vi "Get default PCM configuration_Copy.vi"(11 "PCM Interfaces":T6) -> (2 "Frame Sync Clock Control":T1={"Frame Length"=64, "Frame Sync Pulse Width"=32, "Bit Clock Edge  Sync"=enum."Falling"}, 3 "PCM Data Configuration":T3={"Frame Sync Edge for Channel 0"=enum."Falling", "Channel Count Per Frame"=2, "Channel Length"=32, "Bit Depth"=24, "Channel 0 Offset"=1, "Endianness"=enum."MSB First", "Data Justification"=enum."Left Justified"})   [LabVIEW 2021, in "Audio ADC Shared.lvlib"]
uses:
  Audio ADC Shared.lvlib
  controls/PCM Interface Type_Copy.ctl
  <vilib>/PDM Acquisition Toolkit/shared/controls/PCM Data Format Configuration.ctl
  <vilib>/PDM Acquisition Toolkit/shared/controls/Digital Edge.ctl
  <vilib>/PDM Acquisition Toolkit/shared/controls/PCM Bit Endianness.ctl
  <vilib>/PDM Acquisition Toolkit/shared/controls/PCM Data Justification.ctl
  <vilib>/PDM Acquisition Toolkit/shared/controls/PCM Frame Sync Control.ctl
  <vilib>/PDM Acquisition Toolkit/shared/PDM Shared.lvlib
  controls/Audio ADC Controls.lvlib
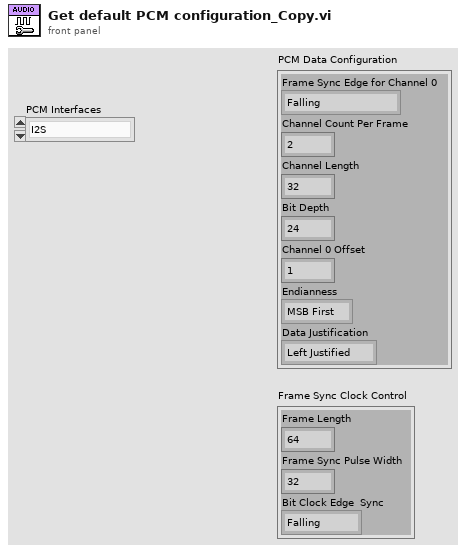
[diagram p1: front panel]
types:
  T1 = typedef "PDM Shared.lvlib/PCM Frame Sync Control.ctl" = cluster{"Frame Length":u16, "Frame Sync Pulse Width":u16, "Bit Clock Edge  Sync":T2}
  T2 = typedef "PDM Shared.lvlib/Digital Edge.ctl" = enum8{"Rising", "Falling"}
  T3 = typedef "PDM Shared.lvlib/PCM Data Format Configuration.ctl" = cluster{"Frame Sync Edge for Channel 0":T2, "Channel Count Per Frame":u8, "Channel Length":u16, "Bit Depth":u8, "Channel 0 Offset":u16, "Endianness":T4, "Data Justification":T5}
  T4 = typedef "PDM Shared.lvlib/PCM Bit Endianness.ctl" = enum16{"MSB First", "LSB First"}
  T5 = typedef "PDM Shared.lvlib/PCM Data Justification.ctl" = enum16{"Left Justified", "Right Justified"}
  T6 = typedef "Audio ADC Controls.lvlib/PCM Interface Type_Copy.ctl" = enum16{"I2S", "Left Justified", "Right Justified", "TDM 4 Channel", "TDM 6 Channel", "TDM 8 Channel", "DSP mode", "DSP mode with 1 bit delay", "PCM Short Frame", "PCM Long Frame"}
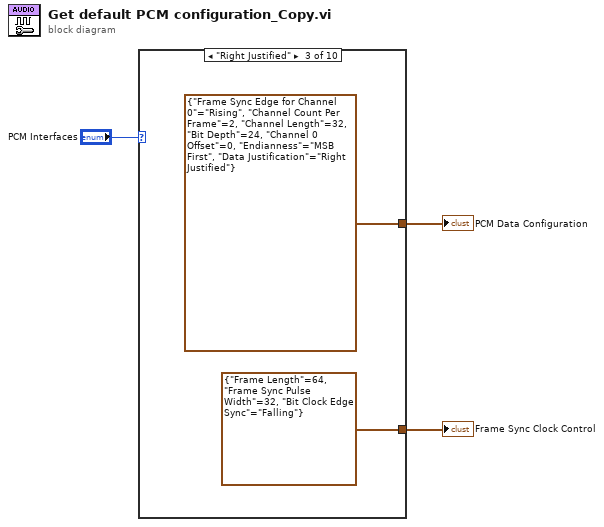
[diagram p0: block diagram]
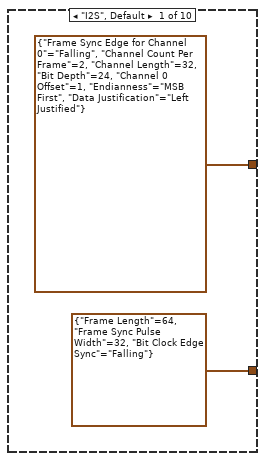
[diagram p2: hidden frame]
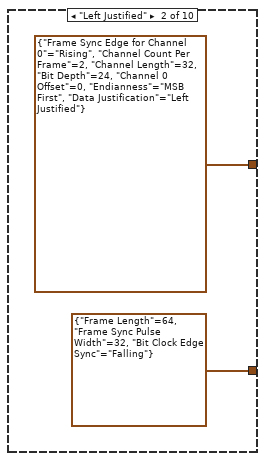
[diagram p3: hidden frame]
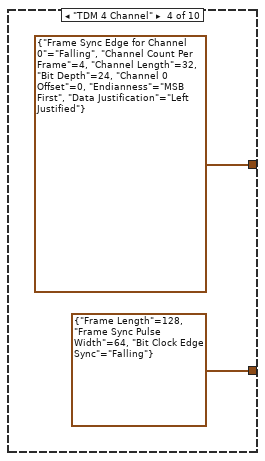
[diagram p4: hidden frame]
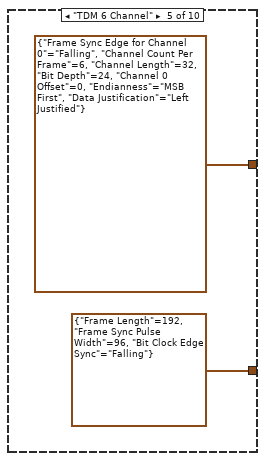
[diagram p5: hidden frame]
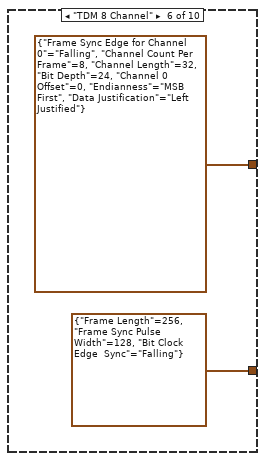
[diagram p6: hidden frame]
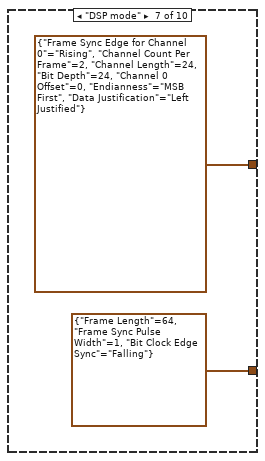
[diagram p7: hidden frame]
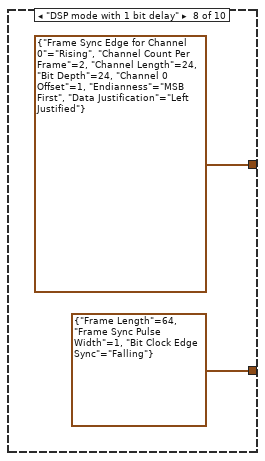
[diagram p8: hidden frame]
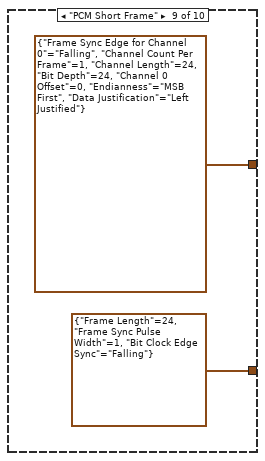
[diagram p9: hidden frame]
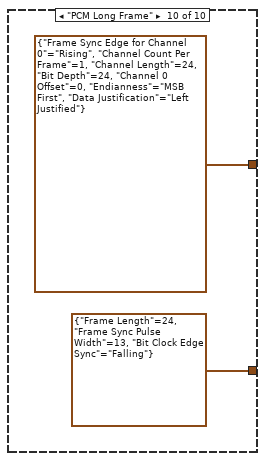
[diagram p10: hidden frame]
diagram:
  n1 = case shown="\"Right Justified\"" "PCM Interfaces" {
    tunnel: [T3 {"Frame Sync Edge for Channel 0"=enum."Falling", "Channel Count Per Frame"=2, "Channel Length"=32, "Bit Depth"=24, "Channel 0 Offset"=1, "Endianness"=enum."MSB First", "Data Justification"=enum."Left Justified"} ("PCM Data Configuration") T3 {"Frame Sync Edge for Channel 0"=enum."Rising", "Channel Count Per Frame"=2, "Channel Length"=32, "Bit Depth"=24, "Channel 0 Offset"=0, "Endianness"=enum."MSB First", "Data Justification"=enum."Left Justified"} ("PCM Data Configuration") T3 {"Frame Sync Edge for Channel 0"=enum."Rising", "Channel Count Per Frame"=2, "Channel Length"=32, "Bit Depth"=24, "Channel 0 Offset"=0, "Endianness"=enum."MSB First", "Data Justification"=enum."Right Justified"} ("PCM Data Configuration") T3 {"Frame Sync Edge for Channel 0"=enum."Falling", "Channel Count Per Frame"=4, "Channel Length"=32, "Bit Depth"=24, "Channel 0 Offset"=0, "Endianness"=enum."MSB First", "Data Justification"=enum."Left Justified"} ("PCM Data Configuration") T3 {"Frame Sync Edge for Channel 0"=enum."Falling", "Channel Count Per Frame"=6, "Channel Length"=32, "Bit Depth"=24, "Channel 0 Offset"=0, "Endianness"=enum."MSB First", "Data Justification"=enum."Left Justified"} ("PCM Data Configuration") T3 {"Frame Sync Edge for Channel 0"=enum."Falling", "Channel Count Per Frame"=8, "Channel Length"=32, "Bit Depth"=24, "Channel 0 Offset"=0, "Endianness"=enum."MSB First", "Data Justification"=enum."Left Justified"} ("PCM Data Configuration") T3 {"Frame Sync Edge for Channel 0"=enum."Rising", "Channel Count Per Frame"=2, "Channel Length"=24, "Bit Depth"=24, "Channel 0 Offset"=0, "Endianness"=enum."MSB First", "Data Justification"=enum."Left Justified"} ("PCM Data Configuration") T3 {"Frame Sync Edge for Channel 0"=enum."Rising", "Channel Count Per Frame"=2, "Channel Length"=24, "Bit Depth"=24, "Channel 0 Offset"=1, "Endianness"=enum."MSB First", "Data Justification"=enum."Left Justified"} ("PCM Data Configuration") T3 {"Frame Sync Edge for Channel 0"=enum."Falling", "Channel Count Per Frame"=1, "Channel Length"=24, "Bit Depth"=24, "Channel 0 Offset"=0, "Endianness"=enum."MSB First", "Data Justification"=enum."Left Justified"} ("PCM Data Configuration") T3 {"Frame Sync Edge for Channel 0"=enum."Rising", "Channel Count Per Frame"=1, "Channel Length"=24, "Bit Depth"=24, "Channel 0 Offset"=0, "Endianness"=enum."MSB First", "Data Justification"=enum."Left Justified"} ("PCM Data Configuration")] -> w2
    tunnel: [T1 {"Frame Length"=64, "Frame Sync Pulse Width"=32, "Bit Clock Edge  Sync"=enum."Falling"} ("Frame Sync Clock Control") T1 {"Frame Length"=64, "Frame Sync Pulse Width"=32, "Bit Clock Edge  Sync"=enum."Falling"} ("Frame Sync Clock Control") T1 {"Frame Length"=64, "Frame Sync Pulse Width"=32, "Bit Clock Edge  Sync"=enum."Falling"} ("Frame Sync Clock Control") T1 {"Frame Length"=128, "Frame Sync Pulse Width"=64, "Bit Clock Edge  Sync"=enum."Falling"} ("Frame Sync Clock Control") T1 {"Frame Length"=192, "Frame Sync Pulse Width"=96, "Bit Clock Edge  Sync"=enum."Falling"} ("Frame Sync Clock Control") T1 {"Frame Length"=256, "Frame Sync Pulse Width"=128, "Bit Clock Edge  Sync"=enum."Falling"} ("Frame Sync Clock Control") T1 {"Frame Length"=64, "Frame Sync Pulse Width"=1, "Bit Clock Edge  Sync"=enum."Falling"} ("Frame Sync Clock Control") T1 {"Frame Length"=64, "Frame Sync Pulse Width"=1, "Bit Clock Edge  Sync"=enum."Falling"} ("Frame Sync Clock Control") T1 {"Frame Length"=24, "Frame Sync Pulse Width"=1, "Bit Clock Edge  Sync"=enum."Falling"} ("Frame Sync Clock Control") T1 {"Frame Length"=24, "Frame Sync Pulse Width"=13, "Bit Clock Edge  Sync"=enum."Falling"} ("Frame Sync Clock Control")] -> w1
    frame "I2S", Default {
    }
    frame "Left Justified" {
    }
    frame "Right Justified" {
    }
    frame "TDM 4 Channel" {
    }
    frame "TDM 6 Channel" {
    }
    frame "TDM 8 Channel" {
    }
    frame "DSP mode" {
    }
    frame "DSP mode with 1 bit delay" {
    }
    frame "PCM Short Frame" {
    }
    frame "PCM Long Frame" {
    }
  }
  "PCM Data Configuration" <- w2
  "Frame Sync Clock Control" <- w1
